vi "FPDAQtoDAQstrings.vi"(1 "front panel":T1={"AO Configuration"=[], "AI Configuration"=[], "Channels: AO"={"Ch"=[], "Amp (V)"=[], "DC (V)"=[], "f (Hz)"=[], "Phase (°)"=[], "Function"=[], "Sweep?"=[]}, "Channels: Lockin"={"Ch"=[13], " f (Hz)"=[], "Phase (°)"=[], "TC (s)"=[0.0], "order"=[0]}, "DAQ Type"=enum."None", "Amplifiers"=enum."Manual", "Gain"=[], "offsets"=[], "Cal Info"=[], "TC (s)"=0.0, "order"=0, "60 Hz prefilter"=FALSE, "LP prefilter"=FALSE, "LP cutoff (Hz)"=0.0, "Fs"=0, "#s"=0} {"AI Configuration"."AI.Coupling" items=["AC"=10045, "DC"=10050, "GND"=10066]; "Channels: AO"."f (Hz)" min=0.001 max=10000.0 format="%.3g"; "Channels: AO"."Phase (°)" format="%.3g"; "Channels: AO"."DC (V)" format="%.3p"; "Channels: AO"."Amp (V)" min=0.0 max=10.0 format="%.3p"; "Channels: Lockin"."order" min=1; "Channels: Lockin"."TC (s)" min=0.0001 format="%#_3p"; "Channels: Lockin"."Phase (°)" format="%.3g"; "Channels: Lockin"."f (Hz)" format="%.3g"; "Cal Info"."SelfCal.LastDate/Time" format="%<%I:%M %p\n%m/%d/%Y>T"}) -> (0 "front panel (DAQmx strings)":T15={"AO Configuration"=[], "AI Configuration"=[], "Channels: AO"={"Ch"=[], "Amp (V)"=[], "DC (V)"=[], "f (Hz)"=[], "Phase (°)"=[], "Function"=[], "Sweep?"=[]}, "Channels: Lockin"={"Ch"=[13], " f (Hz)"=[], "Phase (°)"=[], "TC (s)"=[0.0], "order"=[0]}, "DAQ Type"=enum."None", "Amplifiers"=enum."Manual", "Gain"=[], "offsets"=[], "Cal Info"=[], "TC (s)"=0.0, "order"=0, "60 Hz prefilter"=FALSE, "LP prefilter"=FALSE, "LP cutoff (Hz)"=0.0, "Fs"=0, "#s"=0} {"AI Configuration"."AI.Coupling" items=["AC"=10045, "DC"=10050, "GND"=10066]; "Channels: AO"."f (Hz)" min=0.001 max=10000.0 format="%.3g"; "Channels: AO"."Phase (°)" format="%.3g"; "Channels: AO"."DC (V)" format="%.3p"; "Channels: AO"."Amp (V)" min=0.0 max=10.0 format="%.3p"; "Channels: Lockin"."order" min=1; "Channels: Lockin"."TC (s)" min=0.0001 format="%#_3p"; "Channels: Lockin"."Phase (°)" format="%.3g"; "Channels: Lockin"."f (Hz)" format="%.3g"})   [LabVIEW 2016, in "Lockin.DAQ.lvclass"]
uses:
  Lockin.DAQ.lvclass
  Typedefs/446xAO-enum.ctl
  Typedefs/446xAI-enum.ctl
  Typedefs/AI.coupling-enum.ctl
  Typedefs/AmplifierType-enum.ctl
  Typedefs/DAQType-enum.ctl
  Typedefs/REF-cluster.ctl
  Typedefs/Function-enum.ctl
  Typedefs/AO-cluster.ctl
  Typedefs/Cal Info - Cluster.ctl
  Typedefs/AI.config(UI)-cluster.ctl
  Typedefs/AI.config(UI)-array.ctl
  Typedefs/AO.config(UI)-cluster.ctl
  Typedefs/AO.config(UI)-array.ctl
  Typedefs/Front Panel Cluster.ctl
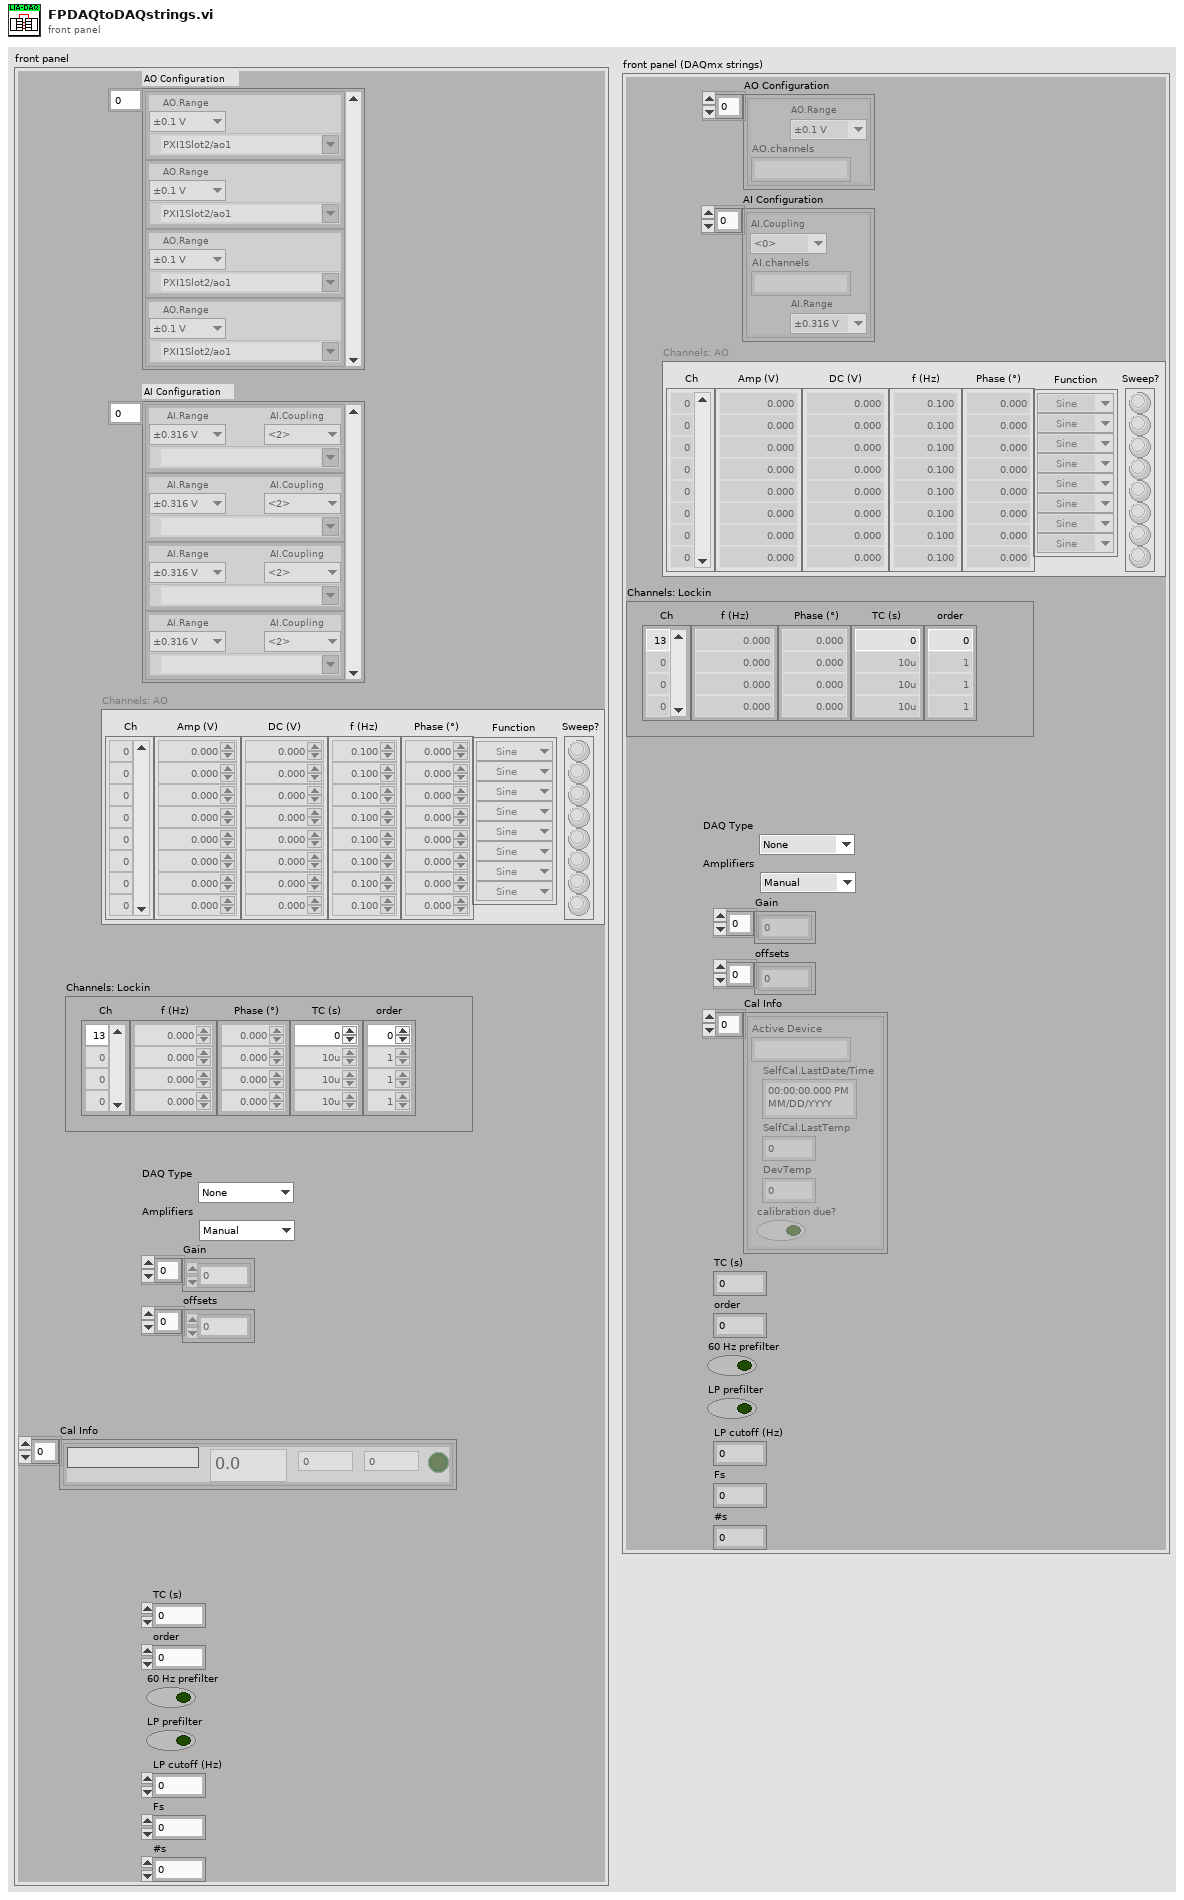
[diagram p1: front panel]
types:
  T1 = typedef "Lockin.DAQ.lvclass/Front Panel Cluster.ctl" = cluster{"AO Configuration":T2, "AI Configuration":T5, "Channels: AO":T9, "Channels: Lockin":T11, "DAQ Type":T12, "Amplifiers":T13, "Gain":dbl[], "offsets":dbl[], "Cal Info":T14[], "TC (s)":dbl, "order":i32, "60 Hz prefilter":bool, "LP prefilter":bool, "LP cutoff (Hz)":dbl, "Fs":i32, "#s":i32}
  T2 = typedef "Lockin.DAQ.lvclass/AO.config(UI)-array.ctl" = T3[]
  T3 = typedef "Lockin.DAQ.lvclass/AO.config(UI)-cluster.ctl" = cluster{"AO.Range":T4, "AO.channels":tag}
  T4 = typedef "Lockin.DAQ.lvclass/446xAO-enum.ctl" = enum16{"±0.1 V", "±1.0 V", "±10.0 V"}
  T5 = typedef "Lockin.DAQ.lvclass/AI.config(UI)-array.ctl" = T6[]
  T6 = typedef "Lockin.DAQ.lvclass/AI.config(UI)-cluster.ctl" = cluster{"AI.Coupling":T7, "AI.channels":tag, "AI.Range":T8}
  T7 = typedef "Lockin.DAQ.lvclass/AI.coupling-enum.ctl" = u16
  T8 = typedef "Lockin.DAQ.lvclass/446xAI-enum.ctl" = enum16{"±0.316 V", "±1.00 V", "±3.16 V", "±10.0 V", "±31.6 V", "±42.4 V"}
  T9 = typedef "Lockin.DAQ.lvclass/AO-cluster.ctl" = cluster{"Ch":i32[], "Amp (V)":dbl[], "DC (V)":dbl[], "f (Hz)":dbl[], "Phase (°)":dbl[], "Function":T10[], "Sweep?":bool[]}
  T10 = typedef "Lockin.DAQ.lvclass/Function-enum.ctl" = enum16{"Sine", "Triangle", "Square", "Sawtooth"}
  T11 = typedef "Lockin.DAQ.lvclass/REF-cluster.ctl" = cluster{"Ch":i32[], " f (Hz)":dbl[], "Phase (°)":dbl[], "TC (s)":dbl[], "order":i32[]}
  T12 = typedef "Lockin.DAQ.lvclass/DAQType-enum.ctl" = enum16{"None", "USB 4431", "PXI 446x"}
  T13 = typedef "Lockin.DAQ.lvclass/AmplifierType-enum.ctl" = enum16{"Manual", "Krohn Hite", "Femto"}
  T14 = typedef "Lockin.DAQ.lvclass/Cal Info - Cluster.ctl" = cluster{"Active Device":string, "SelfCal.LastDate/Time":dbl, "SelfCal.LastTemp":dbl, "DevTemp":dbl, "calibration due?":bool}
  T15 = cluster{"AO Configuration":cluster{"AO.Range":T4, "AO.channels":string}[], "AI Configuration":cluster{"AI.Coupling":T7, "AI.channels":string, "AI.Range":T8}[], "Channels: AO":T9, "Channels: Lockin":T11, "DAQ Type":T12, "Amplifiers":T13, "Gain":dbl[], "offsets":dbl[], "Cal Info":cluster{"Active Device":string, "SelfCal.LastDate/Time":timestamp, "SelfCal.LastTemp":dbl, "DevTemp":dbl, "calibration due?":bool}[], "TC (s)":dbl, "order":i32, "60 Hz prefilter":bool, "LP prefilter":bool, "LP cutoff (Hz)":dbl, "Fs":i32, "#s":i32}
  T16 = cluster{"AI.Coupling":T7, "AI.channels":string, "AI.Range":T8}
  T17 = cluster{"Active Device":string, "SelfCal.LastDate/Time":timestamp, "SelfCal.LastTemp":dbl, "DevTemp":dbl, "calibration due?":bool}
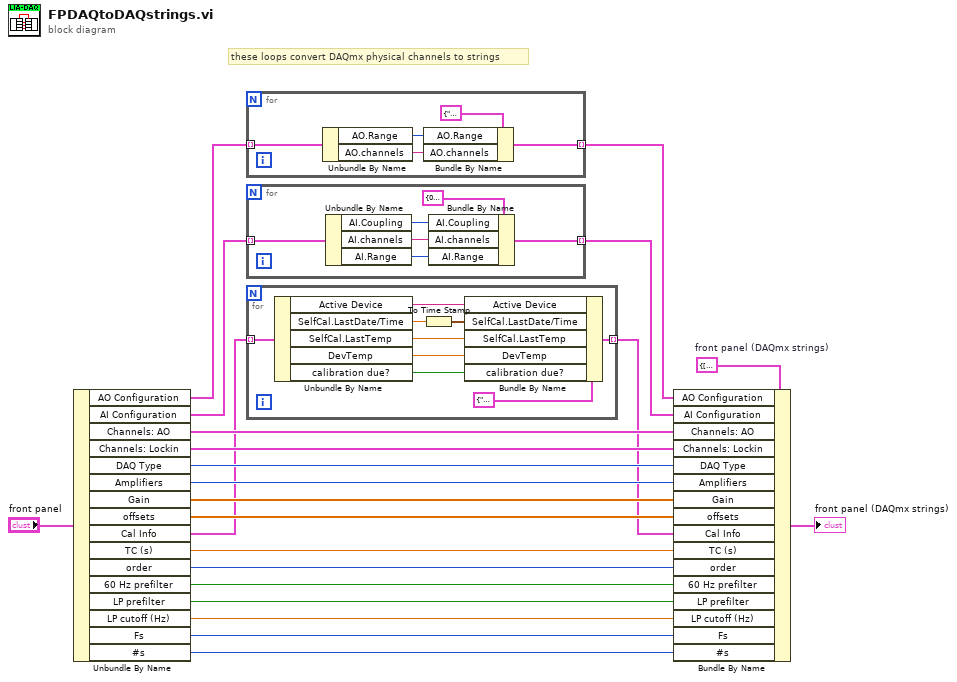
[diagram p0: block diagram]
diagram:
  w22 = T15 {"AO Configuration"=[], "AI Configuration"=[], "Channels: AO"={"Ch"=[], "Amp (V)"=[], "DC (V)"=[], "f (Hz)"=[], "Phase (°)"=[], "Function"=[], "Sweep?"=[]}, "Channels: Lockin"={"Ch"=[13], " f (Hz)"=[], "Phase (°)"=[], "TC (s)"=[0.0], "order"=[0]}, "DAQ Type"=enum."None", "Amplifiers"=enum."Manual", "Gain"=[], "offsets"=[], "Cal Info"=[], "TC (s)"=0.0, "order"=0, "60 Hz prefilter"=FALSE, "LP prefilter"=FALSE, "LP cutoff (Hz)"=0.0, "Fs"=0, "#s"=0}  # front panel (DAQmx strings)
  # "these loops convert DAQmx physical channels to strings"
  n1 = Unbundle By Name("front panel") -> ("AO Configuration"=w20:T2, "AI Configuration"=w19:T5, "Channels: AO"=w18:T9, "Channels: Lockin"=w17:T11, "DAQ Type"=w16:T12, "Amplifiers"=w15:T13, "Gain"=w14:dbl[], "offsets"=w13:dbl[], "Cal Info"=w12:T14[], "TC (s)"=w11:dbl, "order"=w10:i32, "60 Hz prefilter"=w9:bool, "LP prefilter"=w8:bool, "LP cutoff (Hz)"=w7:dbl, "Fs"=w6:i32, "#s"=w5:i32)
  n2 = for {
    tunnel: w20 -> [w27] mode=indexing
    tunnel: [w25] -> w2 mode=indexing
    n3 = Unbundle By Name(w27) -> ("AO.Range"=w26:T4, "AO.channels"=w23:tag)
    n4 = Bundle By Name(cluster=cluster{"AO.Range":T4, "AO.channels":string} {"AO.Range"=enum."±0.1 V", "AO.channels"=""}, "AO.Range"=w26, "AO.channels"=w23) -> (w25:cluster{"AO.Range":T4, "AO.channels":string})
  }
  n5 = for {
    tunnel: w19 -> [w33] mode=indexing
    tunnel: [w32] -> w3 mode=indexing
    n6 = Unbundle By Name(w33) -> ("AI.Coupling"=w28:T7, "AI.channels"=w29:tag, "AI.Range"=w30:T8)
    n7 = Bundle By Name(cluster=T16 {"AI.Coupling"=0, "AI.channels"="", "AI.Range"=enum."±0.316 V"}, "AI.Coupling"=w28, "AI.channels"=w29, "AI.Range"=w30) -> (w32:T16)
  }
  n8 = for {
    tunnel: w12 -> [w41] mode=indexing
    tunnel: [w42] -> w4 mode=indexing
    n9 = Unbundle By Name(w41) -> ("Active Device"=w35:string, "SelfCal.LastDate/Time"=w36:dbl, "SelfCal.LastTemp"=w37:dbl, "DevTemp"=w38:dbl, "calibration due?"=w39:bool)
    n10 = To Time Stamp(1:w36) -> (0:w34:timestamp)
    n11 = Bundle By Name(cluster=T17 {"Active Device"="", "SelfCal.LastDate/Time"=timestamp(0 s since 1904-01-01), "SelfCal.LastTemp"=0.0, "DevTemp"=0.0, "calibration due?"=FALSE}, "Active Device"=w35, "SelfCal.LastDate/Time"=w34, "SelfCal.LastTemp"=w37, "DevTemp"=w38, "calibration due?"=w39) -> (w42:T17)
  }
  n12 = Bundle By Name(cluster=w22, "AO Configuration"=w2, "AI Configuration"=w3, "Channels: AO"=w18, "Channels: Lockin"=w17, "DAQ Type"=w16, "Amplifiers"=w15, "Gain"=w14, "offsets"=w13, "Cal Info"=w4, "TC (s)"=w11, "order"=w10, "60 Hz prefilter"=w9, "LP prefilter"=w8, "LP cutoff (Hz)"=w7, "Fs"=w6, "#s"=w5) -> (→"front panel (DAQmx strings)":T15)
